vi "Set Motor Power.vi"(10 "Cluster":T1) -> ()   [LabVIEW 2013]
uses:
  Drive Train Metrics.ctl
  CmdFlag.ctl
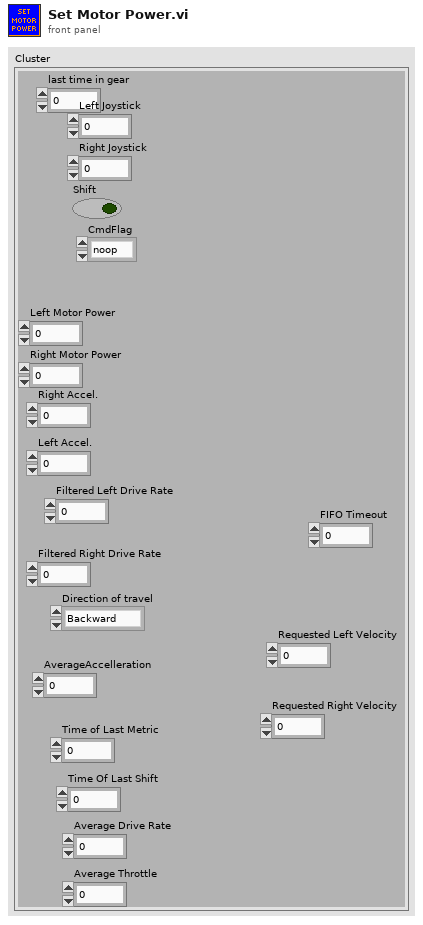
[diagram p1: front panel]
types:
  T1 = typedef "Drive Train Metrics.ctl" = cluster{"last time in gear":u32, "Shift":bool, "Right Joystick":dbl, "Left Joystick":dbl, "CmdFlag":T2, "Right Motor Power":dbl, "Left Motor Power":dbl, "Right Accel.":dbl, "Left Accel.":dbl, "Filtered Left Drive Rate":dbl, "Filtered Right Drive Rate":dbl, "Direction of travel":enum16{"Backward", "Forward", "Spin"}, "AverageAccelleration":dbl, "Time of Last Metric":u32, "Time Of Last Shift":dbl, "Average Drive Rate":dbl, "Average Throttle":dbl, "FIFO Timeout":i32, "Requested Left Velocity":dbl, "Requested Right Velocity":dbl}
  T2 = typedef "CmdFlag.ctl" = enum16{"noop", "suspend", "resume"}
  T3 = typedef "WPI_MotorControlDeviceRef.ctl" = cluster{"DeviceStatus":errorcluster, "Type":enum16{"PWM", "CAN"}, "PWM":cluster{"Digital Module":T4, "PWM Channel":T5, "DeadBand":T6}, "CAN":cluster{"Device Number":u8, "Control Mode":T7, "Semaphore":T8, "Max Vout":dbl}, "Invert":bool, "TransformRef":T9, "InvTransformRef":T9}
  T4 = typedef "FPGA_TypedefDigitalModule.ctl" = enum16{"Digital Module 1", "Digital Module 2"}
  T5 = typedef "FPGA_DIOPWMChannel.ctl" = enum8{"PWM 1", "PWM 2", "PWM 3", "PWM 4", "PWM 5", "PWM 6", "PWM 7", "PWM 8", "PWM 9", "PWM 10", "Invalid"}
  T6 = typedef "WPI_PWMDeadband.ctl" = cluster{"Name":string, "maxPositivePwm":i32, "minPositivePwm":i32, "centerPwm":i32, "maxNegativePwm":i32, "minNegativePwm":i32, "angularRange":u16}
  T7 = typedef "WPI_CANJaguar_ControlMode.ctl" = enum8{"Percent VBus", "Current", "Speed", "Position", "Voltage"}
  T8 = typedef "Semaphore RefNum" = refnum<k1>
  T9 = typedef "WPI_PWMTransform_ConPane.ctl" = refnum<vi>
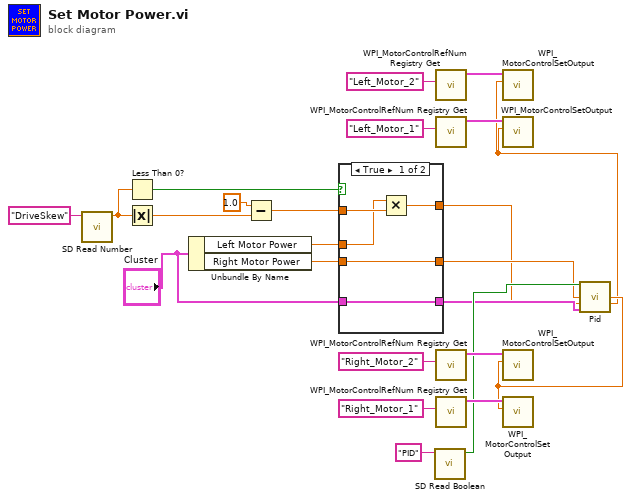
[diagram p0: block diagram]
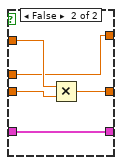
[diagram p2: hidden frame]
diagram:
  n1 = call <vilib>:"SD Read Number.vi"("Name"="DriveSkew") -> ("Numeric"=w14:dbl)  [unwired: 8 in, 2 out]
  n2 = Less Than 0?(x=w14) -> (x < 0?=w15:bool)
  n3 = Absolute Value(x=w14) -> (abs(x)=w12:dbl)
  n4 = Unbundle By Name("Cluster") -> ("Left Motor Power"=w10:dbl, "Right Motor Power"=w9:dbl)
  n5 = Subtract(x=1.0, y=w12) -> (x-y=w11:dbl)
  n6 = case shown="True" w15 {
    tunnel: [w28 w32] -> w3
    tunnel: [w27 w34] -> w4
    tunnel: w11 -> [w29 w33]
    tunnel: w10 -> [w26 w32]
    tunnel: w9 -> [w27 w31]
    tunnel: "Cluster" -> [w25 w30]
    tunnel: [w25 w30] -> w5
    frame True {
      n7 = Multiply(x=w26, y=w29) -> (x*y=w28:dbl)
    }
    frame False {
      n8 = Multiply(x=w33, y=w31) -> (x*y=w34:dbl)
    }
  }
  n9 = call <vilib>:"SD Read Boolean.vi"("Name"="PID") -> ("Boolean"=w6:bool)  [unwired: 8 in, 2 out]
  n10 = call <vilib>:"WPI_MotorControlRefNum Registry Get.vi"("refnum name"="Left_Motor_2") -> ("MotorControlDevRef"=w24:T3)  [unwired: 9 in, 1 out]
  n11 = call <vilib>:"WPI_MotorControlRefNum Registry Get.vi"("refnum name"="Left_Motor_1") -> ("MotorControlDevRef"=w21:T3)  [unwired: 9 in, 1 out]
  n12 = call <vilib>:"WPI_MotorControlRefNum Registry Get.vi"("refnum name"="Right_Motor_2") -> ("MotorControlDevRef"=w19:T3)  [unwired: 9 in, 1 out]
  n13 = call <vilib>:"WPI_MotorControlRefNum Registry Get.vi"("refnum name"="Right_Motor_1") -> ("MotorControlDevRef"=w17:T3)  [unwired: 9 in, 1 out]
  n14 = call "Pid.vi"("Boolean"=w6, "Right Motor Power"=w4, "Left Motor Power"=w3, "Cluster"=w5) -> ("Right Motor Output"=w2:dbl, "Left Motor Output"=w1:dbl)  [unwired: 10 in]
  n15 = call <vilib>:"WPI_MotorControlSetOutput.vi"("Output"=w1, "MotorControlDevRef"=w24) -> ()  [unwired: 7 in, 3 out]
  n16 = call <vilib>:"WPI_MotorControlSetOutput.vi"("Output"=w1, "MotorControlDevRef"=w21) -> ()  [unwired: 7 in, 3 out]
  n17 = call <vilib>:"WPI_MotorControlSetOutput.vi"("Output"=w2, "MotorControlDevRef"=w19) -> ()  [unwired: 7 in, 3 out]
  n18 = call <vilib>:"WPI_MotorControlSetOutput.vi"("Output"=w2, "MotorControlDevRef"=w17) -> ()  [unwired: 7 in, 3 out]
